vi "gotowoscDoPomiaru.vi"(3 "Wczytaj_zapisz":T2, 5 "Gotowoœæ":T1) -> (2 "Gotowoœæ wyjœcie":T1)   [LabVIEW 2014]
uses:
  gotowoscDoPomiaruVIs/Gotowosc.ctl
  gotowoscDoPomiaruVIs/wczytaj_zapisz.ctl
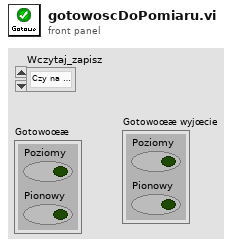
[diagram p1: front panel]
types:
  T1 = typedef "Gotowosc.ctl" = cluster{"Poziomy":bool, "Pionowy":bool}
  T2 = typedef "wczytaj_zapisz.ctl" = enum16{"Czy na pozycjach?", "Zapisz", "Wczytaj"}
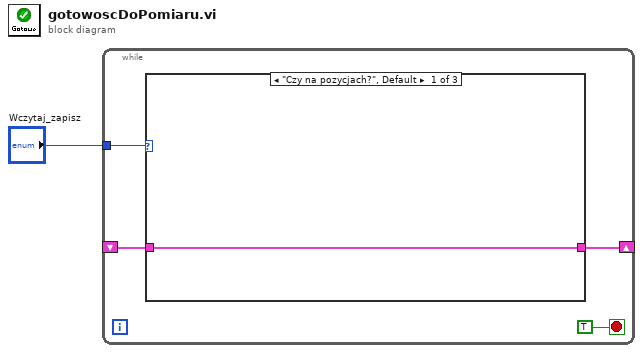
[diagram p0: block diagram]
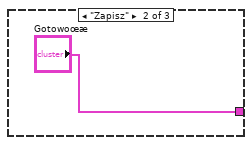
[diagram p2: hidden frame]
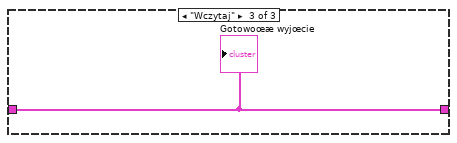
[diagram p3: hidden frame]
diagram:
  n1 = while {
    tunnel: "Wczytaj_zapisz" -> [w4]
    shift-right: [w2] -> _
    shift-left: _ -> [w3]
    stop <- TRUE stop-if-true
    n2 = case shown="\"Czy na pozycjach?\", Default" w4 {
      tunnel: w3 -> [w6 _ w8]
      tunnel: [w6 "Gotowoœæ" w8] -> w2
      frame "Czy na pozycjach?", Default {
      }
      frame "Zapisz" {
      }
      frame "Wczytaj" {
        "Gotowoœæ wyjœcie" <- w8
      }
    }
  }
